vi "Power Meter (No Objects).vi"(8 "error in (no error)":errorcluster, 11 "VISA resource name":refnum<visa-resource-name>) -> (0 "error out":errorcluster, 3 "Power Meter Out":T2 {"Averaging Points" format="%.2f"; "Filter" items=["Orange"=1, "Green"=2, "Yellow"=3]})   [LabVIEW 2013]
uses:
  Public/Filters.ctl
  Newport 1830-C.lvlib
panel:
  out "Status":string
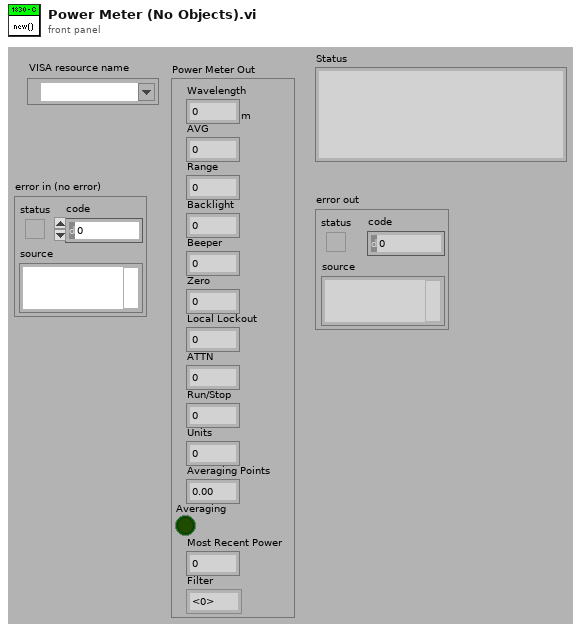
[diagram p1: front panel]
types:
  T1 = typedef "Newport 1830-C.lvlib/Filters.ctl" = u16
  T2 = cluster{"Wavelength":dbl[unit], "AVG":u16, "Range":u16, "Backlight":u16, "Beeper":u16, "Zero":u16, "Local Lockout":u16, "ATTN":u16, "Run/Stop":u16, "Units":u16, "Averaging Time":dbl, "Averaging":bool, "Most Recent Power":dbl, "Filter":T1}
  T3 = cluster{"Wavelength":dbl[unit], "AVG":u16, "Range":u16, "Backlight":u16, "Beeper":u16, "Zero":u16, "Local Lockout":u16, "ATTN":u16, "Run/Stop":u16, "Units":u16, "Averaging Time":u32, "Averaging":bool, "Most Recent Power":dbl, "Filter":T1}
  T4 = cluster{"Wavelength":dbl[unit], "AVG":u16, "Range":u16, "Backlight":u16, "Beeper":u16, "Zero":u16, "Local Lockout":u16, "ATTN":u16, "Run/Stop":u16, "Units":u16, "Averaging Points":u32, "Averaging":bool, "Most Recent Power":dbl, "Filter":T1}
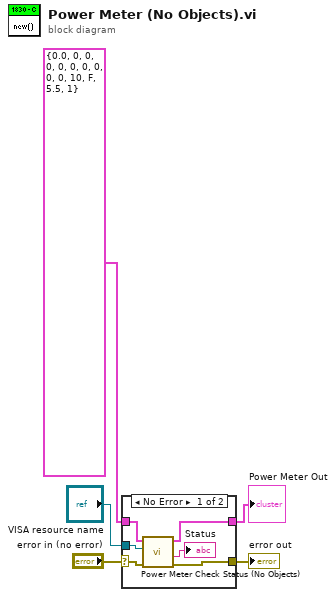
[diagram p0: block diagram]
diagram:
  n1 = case shown="No Error" "error in (no error)" {
    selector: "error in (no error)" -> [w9 w13]
    tunnel: [w8 w13] -> w4
    tunnel: [w7 w12] -> w2
    tunnel: T3 {"Wavelength"=0.0, "AVG"=0, "Range"=0, "Backlight"=0, "Beeper"=0, "Zero"=0, "Local Lockout"=0, "ATTN"=0, "Run/Stop"=0, "Units"=0, "Averaging Time"=10, "Averaging"=FALSE, "Most Recent Power"=5.5, "Filter"=1} ("Cluster of class private data") -> [w10 w12]
    tunnel: "VISA resource name" -> [w6 _]
    frame No Error {
      n2 = call "Power Meter Check Status (No Objects).vi"("error in (no error)"=w9, "VISA resource name"=w6, "Cluster In"=w10) -> ("error out"=w8:errorcluster, "Status"=→"Status":string, "Cluster Out"=w7:T4)  [unwired: 6 in]
    }
    frame Error {
    }
  }
  "error out" <- w4
  "Power Meter Out" <- w2
